vi "K2182A_Check_Queue.vi"(7 "error in (no error)":errorcluster, 10 "queue":refnum<queue>) -> (0 "error out":errorcluster, 1 "Control":T1, 3 "New Entries?":bool)   [LabVIEW 2019]
uses:
  K2812A/K2812A_control.ctl
  Equipment/Keithley 622x/Configure/2182 -A/Low Level/Typedefs/KE2182 -- Voltage Ranges.ctl
  Equipment/Keithley 622x/Keithley 622x.lvlib
panel:
  out "Numeric":i32
  # "K 2182A"
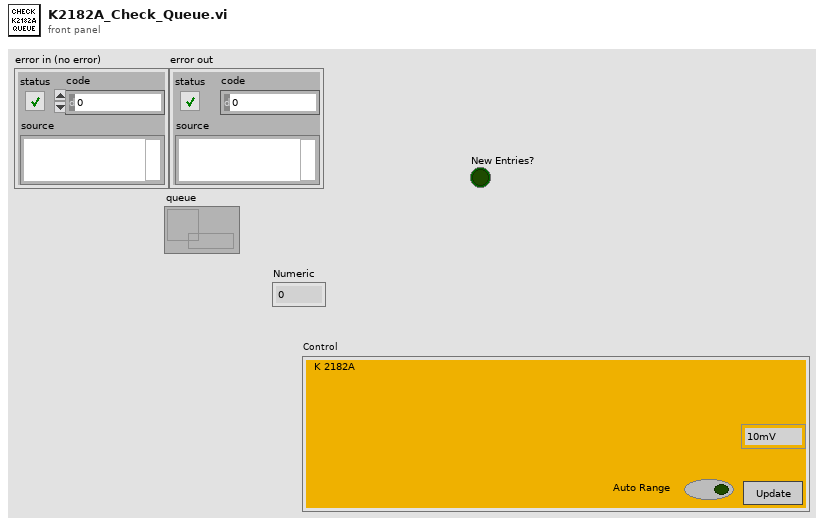
[diagram p1: front panel]
types:
  T1 = typedef "K2812A_control.ctl" = cluster{"Update":bool, "Range selector":T2, "Auto Range":bool}
  T2 = typedef "Keithley 622x.lvlib/KE2182 -- Voltage Ranges.ctl" = enum16{"10mV", "100mV", "1V", "10V", "100V"}
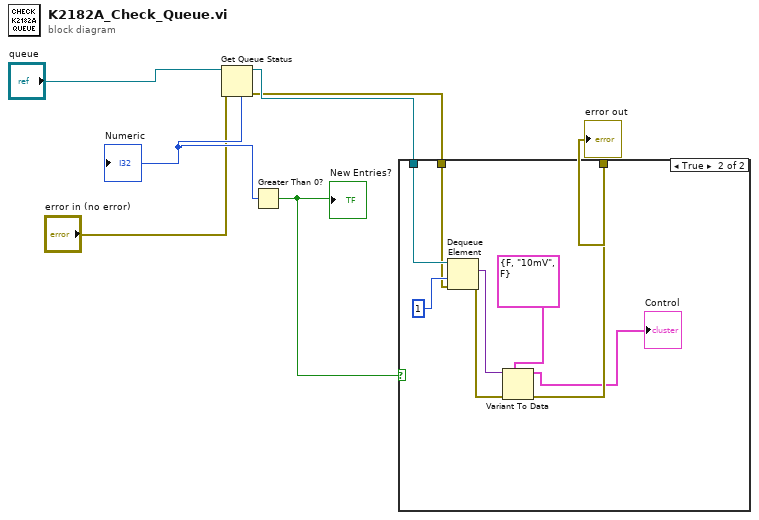
[diagram p0: block diagram]
diagram:
  n1 = Get Queue Status(queue="queue", error in (no error)="error in (no error)") -> (queue out=w6:refnum<queue>, error out=w4:errorcluster, # elements in queue=w7:i32)  [unwired: 1 in, 5 out]
  "Numeric" <- w7
  n2 = Greater Than 0?(x=w7) -> (x > 0?=w5:bool)
  "New Entries?" <- w5
  n3 = case shown="True" w5 {
    tunnel: w6 -> [_ w14]
    tunnel: w4 -> [w8 w13]
    tunnel: [w8 w11] -> w2
    frame False {
    }
    frame True {
      n4 = Dequeue Element(queue=w14, timeout in ms (-1)=1, error in (no error)=w13) -> (element=w15:variant, error out=w12:errorcluster)  [unwired: 2 out]
      n5 = Variant To Data(error in=w12, type=T1 {"Update"=FALSE, "Range selector"=enum."10mV", "Auto Range"=FALSE} ("K2182A Cluster 2"), Variant=w15) -> (data=→"Control":T1, error out=w11:errorcluster)
    }
  }
  "error out" <- w2
